vi "context use private key.vi"(8 "error in":errorcluster, 9 "format":i32, 10 "certificate data":string, 11 "connector":u64) -> (0 "error out":errorcluster)   [LabVIEW 2016, in "async tls dl.lvlib"]
uses:
  async tls dl.lvlib
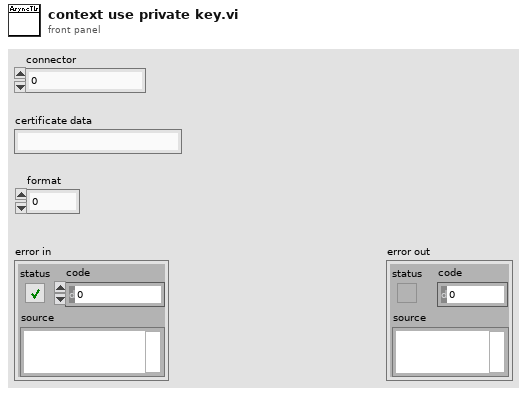
[diagram p1: front panel]
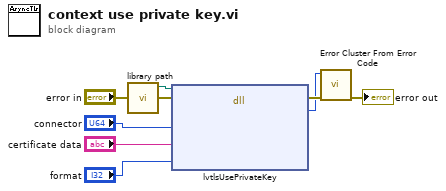
[diagram p0: block diagram]
diagram:
  n1 = call "library path.vi"() -> ("path"=w1:path)  [unwired: 11 in]
  n2 = dll-call lib="C:/Users/IEUser/Desktop/libasynclvtls/lvasynctls.dll" fn="lvtlsUsePrivateKey"(path in=w1, error in="error in", "connCreator"="connector", "certificate"="certificate data", "format"="format") -> (error out=w8:errorcluster, "err"=w7:i32)  [unwired: 4 in, 1 out]
  n3 = call <vilib>:"Error Cluster From Error Code.vi"("error in (no error)"=w8, "error code (0)"=w7) -> ("error out"=→"error out":errorcluster)  [unwired: 7 in]
